vi "Search for Frame in Frames.vi"(9 "Frame Name":string, 11 "Frame Names":string[](array[string])) -> (3 "index of element":i32)   [LabVIEW 2020]
uses:
  <userlib>/_OpenG.lib/string/string.llb/openg_string.lvlib
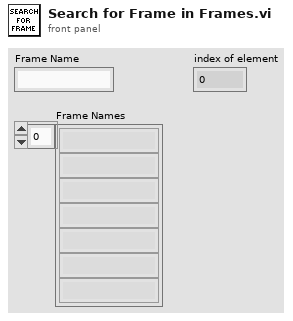
[diagram p1: front panel]
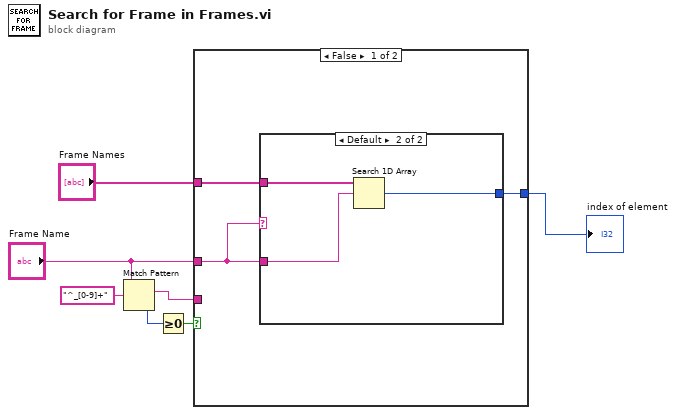
[diagram p0: block diagram]
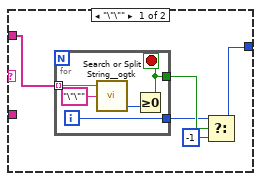
[diagram p2: hidden frame]
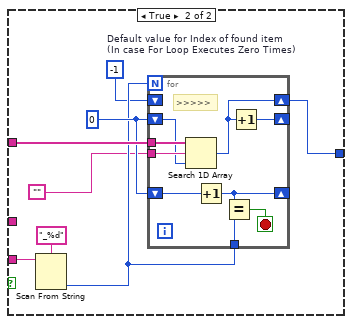
[diagram p3: hidden frame]
diagram:
  n1 = Match Pattern(string="Frame Name", regular expression="^_[0-9]+") -> (match substring=w1:string, offset past match=w3:i32)  [unwired: 1 in, 2 out]
  n2 = Greater Or Equal To 0?(x=w3) -> (x >= 0?=w2:bool)
  n3 = case shown="False" w2 {
    tunnel: "Frame Names" -> [w10 w31]
    tunnel: [w9 w24] -> w6
    tunnel: "Frame Name" -> [w8 _]
    tunnel: w1 -> [_ w30]
    frame False {
      n4 = case shown="Default" w8 {
        tunnel: w10 -> [w12 w23]
        tunnel: w8 -> [_ w22]
        tunnel: [w11 w21] -> w9
        frame "\"\"" {
          n5 = for {
            tunnel: w12 -> [w20] mode=indexing
            tunnel: [w16] -> w15
            tunnel: [w17] -> w14
            i -> [w17]
            stop <- w16 stop-if-true
            n6 = call <userlib>:"Search or Split String__ogtk.vi"("search string/char (-)"="\"\"", "string"=w20) -> ("offset after match"=w18:i32)  [unwired: 1 in, 2 out]
            n7 = Greater Or Equal To 0?(x=w18) -> (x >= 0?=w16:bool)
          }
          n8 = Select(t=w14, s=w15, f=-1) -> (s? t:f=w11:i32)
        }
        frame Default {
          n9 = Search 1D Array(1D array=w23, element=w22) -> (index of element=w21:i32)  [unwired: 1 in]
        }
      }
    }
    frame True {
      w25 = -1  # Default value for Index of found item (In case For Loop Executes Zero Times)
      w28 = 0
      n10 = Scan From String(format string="_%d", input string=w30) -> (output 1=w27:i32)  [unwired: 3 in, 3 out]
      n11 = for {
        N: w27 -> [_]
        tunnel: w31 -> [w40]
        tunnel: "" -> [w39]
        shift-right: [w38] -> _
        shift-left: w28 -> [w37]
        shift-right: [w35] -> _
        shift-left: w28 -> [w36]
        tunnel: w27 -> [w34]
        shift-right: [w32] -> w24
        shift-left: w25 -> [_]
        stop <- w33 stop-if-true
        # ">>>>>"
        n12 = Search 1D Array(1D array=w40, element=w39, start index (0)=w37) -> (index of element=w32:i32)
        n13 = Increment(x=w36) -> (x+1=w35:i32)
        n14 = Equal?(x=w35, y=w34) -> (x = y?=w33:bool)
        n15 = Increment(x=w32) -> (x+1=w38:i32)
      }
    }
  }
  "index of element" <- w6
